vi "Set Report Font.vi"(0 "report in":refnum<class "NI_Word.lvclass">, 1 "text color (unchanged)":u32(colorbox)=16777216, 2 "font settings source":u16(ring) items=["VI Inputs", "Font Dialog Box"], 5 "text options":T2, 9 "font settings":T3={"Charset (-1)"=-1, "Weight (-1)"=-1, "Name"="", "Size"=" "}, 11 "error in (no error)":errorcluster) -> (4 "report out":refnum<class "NI_Word.lvclass">, 6 "font out":T1={"font name"="", "font size"=0.0, "bold"=0, "italic"=0, "underline"=0, "strike through"=0, "font color"=16777216} {"font size" format="%0.2f"; "strike through" items=["Unchanged", "Yes", "No"]; "underline" items=["Unchanged", "Yes", "No"]; "italic" items=["Unchanged", "Yes", "No"]; "bold" items=["Unchanged", "Yes", "No"]}, 15 "error out":errorcluster)   [LabVIEW 2020, in "NI_Word.lvclass"]
doc: "Sets the font properties of the report, including those in the headers and footers."
uses:
  <vilib>/Utility/NIReport.llb/Word/NI_Word.lvclass
  <vilib>/addons/_office/_exclsub.llb/font.ctl
  <vilib>/Utility/NIReport.llb/Word/NI_Word.lvclass/NI_Word.ctl
  <vilib>/addons/_office/NI_ReportGenerationToolkit.lvlib
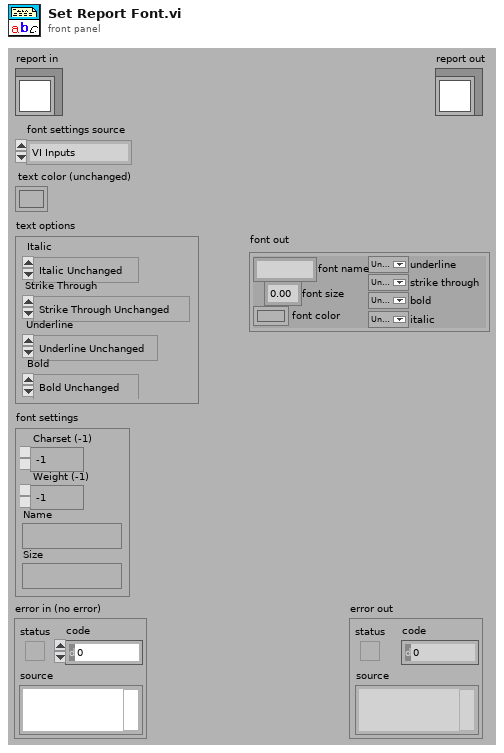
[diagram p1: front panel]
types:
  T1 = typedef "NI_ReportGenerationToolkit.lvlib/font.ctl" = cluster{"font name":string, "font size":dbl, "bold":u16, "italic":u16, "underline":u16, "strike through":u16, "font color":u32}
  T2 = cluster{"Italic":enum16{"Italic Unchanged", "Italic On", "Italic Off"}, "Strike Through":enum16{"Strike Through Unchanged", "Strike Through On", "Strike Through Off"}, "Underline":enum16{"Underline Unchanged", "Underline On", "Underline Off"}, "Bold":enum16{"Bold Unchanged", "Bold On", "Bold Off"}}
  T3 = cluster{"Charset (-1)":i16, "Weight (-1)":i16, "Name":string, "Size":string}
  T4 = typedef "NI_ReportGenerationCore.lvlib/Report Data Members.ctl" = cluster{"font":T5, "from template?":bool}
  T5 = typedef "NI_ReportGenerationCore.lvlib/font.ctl" = cluster{"font name":string, "font size":dbl, "bold":u16, "italic":u16, "underline":u16, "strike through":u16, "font color":u32}
  T6 = enum16{"Italic Unchanged", "Italic On", "Italic Off"}
  T7 = enum16{"Underline Unchanged", "Underline On", "Underline Off"}
  T8 = enum16{"Strike Through Unchanged", "Strike Through On", "Strike Through Off"}
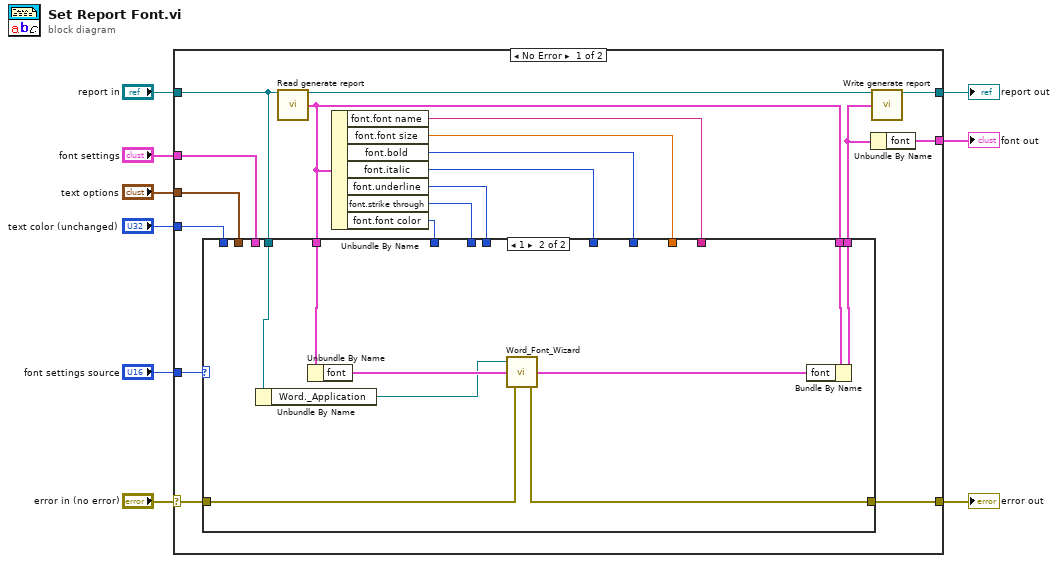
[diagram p0: block diagram]
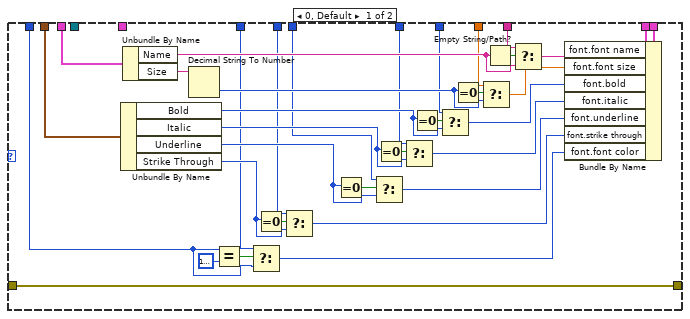
[diagram p2: hidden frame]
diagram:
  n1 = case shown="No Error" "error in (no error)" {
    selector: "error in (no error)" -> [w19 w74]
    tunnel: [w18 w74] -> w8
    tunnel: [w12 w73] -> w6
    tunnel: "report in" -> [w10 w73]
    tunnel: "font settings source" -> [w21 _]
    tunnel: "font settings" -> [w20 _]
    tunnel: "text options" -> [w17 _]
    tunnel: "text color (unchanged)" -> [w16 _]
    tunnel: [w15 _] -> w1
    frame No Error {
      n2 = call-dynamic "Read generate report.vi"("report in"=w10) -> ("report out"=w13:refnum<class "NI_Word.lvclass">, "generate report"=w14:T4)  [unwired: 12 in, 1 out]
      n3 = Unbundle By Name(w14) -> ("font.font name"=w22:string, "font.font size"=w23:dbl, "font.bold"=w24:u16, "font.italic"=w25:u16, "font.underline"=w28:u16, "font.strike through"=w27:u16, "font.font color"=w26:u32)
      n4 = case shown="1" w21 {
        tunnel: w17 -> [w63 _]
        tunnel: w20 -> [w62 _]
        tunnel: w22 -> [w59 _]
        tunnel: w23 -> [w56 _]
        tunnel: w24 -> [w52 _]
        tunnel: w25 -> [w47 _]
        tunnel: w26 -> [w43 _]
        tunnel: w16 -> [w42 _]
        tunnel: w27 -> [w40 _]
        tunnel: w14 -> [_ w72]
        tunnel: w14 -> [w32 w69]
        tunnel: [w31 w68] -> w11
        tunnel: w28 -> [w30 _]
        tunnel: w19 -> [w29 w67]
        tunnel: [w29 w66] -> w18
        tunnel: w10 -> [_ w65]
        frame 0, Default {
          n5 = Unbundle By Name(w63) -> ("Bold"=w53:enum16{"Bold Unchanged", "Bold On", "Bold Off"}, "Italic"=w50:T6, "Underline"=w48:T7, "Strike Through"=w45:T8)
          n6 = Unbundle By Name(w62) -> ("Name"=w58:string, "Size"=w61:string)
          n7 = Decimal String To Number(string=w61) -> (number=w55:i32)  [unwired: 3 out]
          n8 = Equal?(x=w42, y=u32 16777216) -> (x = y?=w44:bool)
          n9 = Select(t=w43, s=w44, f=w42) -> (s? t:f=w33:u32)
          n10 = Equal To 0?(x=w45) -> (x = 0?=w46:bool)
          n11 = Select(t=w40, s=w46, f=w45) -> (s? t:f=w34:u16)
          n12 = Equal To 0?(x=w48) -> (x = 0?=w49:bool)
          n13 = Select(t=w30, s=w49, f=w48) -> (s? t:f=w35:u16)
          n14 = Equal To 0?(x=w50) -> (x = 0?=w51:bool)
          n15 = Select(t=w47, s=w51, f=w50) -> (s? t:f=w36:u16)
          n16 = Equal To 0?(x=w53) -> (x = 0?=w54:bool)
          n17 = Select(t=w52, s=w54, f=w53) -> (s? t:f=w37:u16)
          n18 = Equal To 0?(x=w55) -> (x = 0?=w57:bool)
          n19 = Select(t=w56, s=w57, f=w55) -> (s? t:f=w38:dbl)
          n20 = Empty String/Path?(string/path=w58) -> (empty?=w60:bool)
          n21 = Select(t=w59, s=w60, f=w58) -> (s? t:f=w39:string)
          n22 = Bundle By Name(cluster=w32, "font.font name"=w39, "font.font size"=w38, "font.bold"=w37, "font.italic"=w36, "font.underline"=w35, "font.strike through"=w34, "font.font color"=w33) -> (w31:T4)
        }
        frame 1 {
          n23 = Unbundle By Name(w65) -> ("Word._Application"=w64:refnum<k7>)
          n24 = Unbundle By Name(w72) -> ("font"=w71:T5)
          n25 = call <vilib>:"Word_Font_Wizard.vi"("error in (no error)"=w67, "font in"=w71, "Word._Application"=w64) -> ("error out"=w66:errorcluster, "font out"=w70:T1)  [unwired: 1 out]
          n26 = Bundle By Name(cluster=w69, "font"=w70) -> (w68:T4)
        }
      }
      n27 = Unbundle By Name(w11) -> ("font"=w15:T5)
      n28 = call-dynamic "Write generate report.vi"("report in"=w13, "generate report"=w11) -> ("report out"=w12:refnum<class "NI_Word.lvclass">)  [unwired: 12 in, 1 out]
    }
    frame Error {
    }
  }
  "error out" <- w8
  "report out" <- w6
  "font out" <- w1
